vi "d1000 start sa move.vi"(6 "Tacc":dbl, 7 "MaxVel":i32, 9 "StrVel":i32, 10 "Pos":i32, 11 "axis":i16) -> (3 "function return":u32)   [LabVIEW 2019, in "Dmc1000.lvlib"]
doc: "DMC1000_API DWORD WINAPI d1000_start_sa_move(short axis,long Pos, long StrVel,long MaxVel,double Tacc);"
uses:
  Dmc1000.lvlib
  Dmc1000.dll
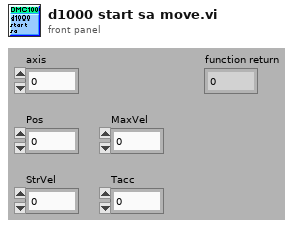
[diagram p1: front panel]
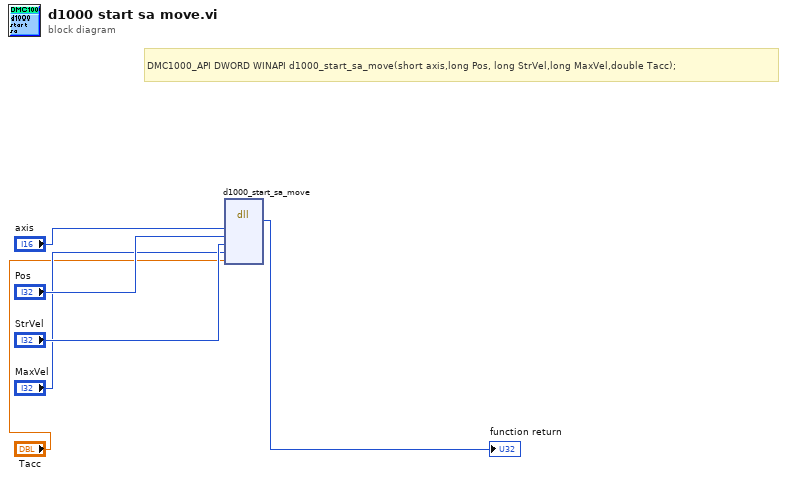
[diagram p0: block diagram]
diagram:
  # "DMC1000_API DWORD WINAPI d1000_start_sa_move(short axis,long Pos, long StrVel,long MaxVel,double Tacc);"
  n1 = dll-call lib="C:/Users/VIC/Desktop/Standar Program/System/LLB/DMC1000B/Dmc1000.dll" fn="d1000_start_sa_move" ("Dmc1000.dll:_d1000_start_sa_move@24")("axis"="axis", "Pos"="Pos", "StrVel"="StrVel", "MaxVel"="MaxVel", "Tacc"="Tacc") -> ("return type"=→"function return":u32)  [unwired: 8 in, 2 out]
